vi "SFCS_ChkRoute_ComCode.vi"(5 "URL":string) -> (1 "Status":string)   [LabVIEW 2011]
uses:
  Instance           4 29Saved   SFCS_ChkRoute_ComCode .vi
  Instance           1 29Saved   SFCS_ChkRoute_ComCode .vi
  Instance           2 29Saved   SFCS_ChkRoute_ComCode .vi
  Instance           3 29Saved   SFCS_ChkRoute_ComCode .vi
  Instance           5 29Saved   SFCS_ChkRoute_ComCode .vi
  data/MCSDLL.dll
panel:
  out "軟體版本Software Version":string
  out "Begin time":u32
  out "SFCS System Enable":string
  out "ComCode":string
  out "Category":string
  out "COMCODE":string
  out "STAGE":string
  out "Unit SN":string
  out "USN_Length":i32
  out "SFCS_IP":string
  # "SFCS Check Route"
  # "2014-12-15"
  # "SFCS的網址"
  # "站名"
  # "序號"
  # "訊息"
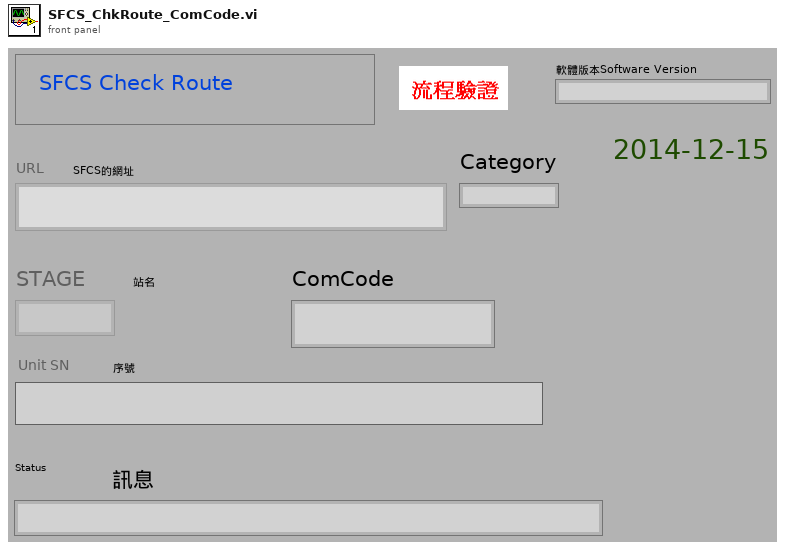
[diagram p1: front panel]
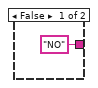
[diagram p5: hidden frame]
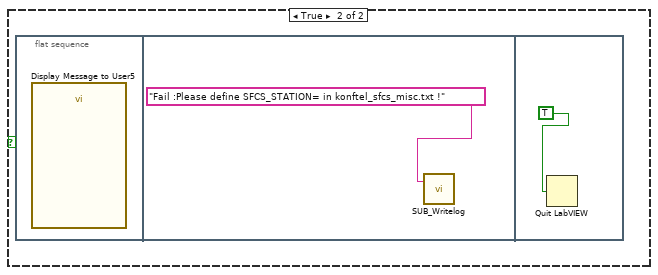
[diagram p7: hidden frame]
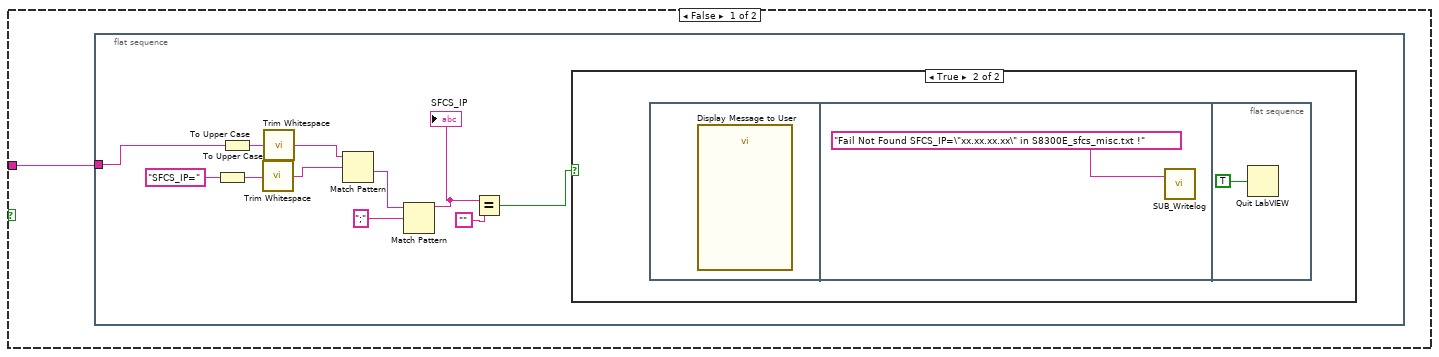
[diagram p9: hidden frame]
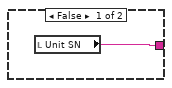
[diagram p11: hidden frame]
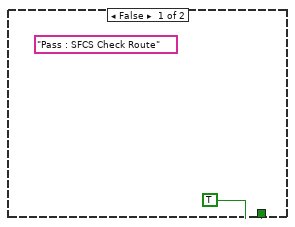
[diagram p12: hidden frame]
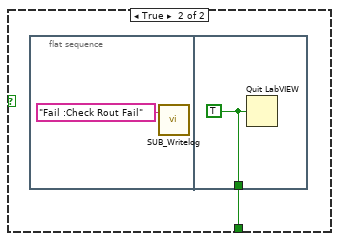
[diagram p13: hidden frame]
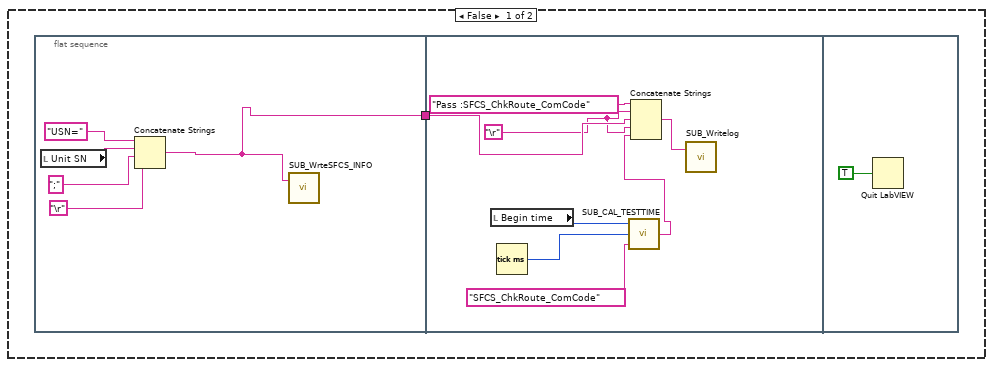
[diagram p14: hidden frame]
diagram:
  n1 = flat-sequence {
    tunnel: [w120] -> w2
    tunnel: [w119] -> w1
    tunnel: w2 -> [w139]
    tunnel: w1 -> [w135]
    frame #0 {
      n2 = Tick Count (ms)() -> (millisecond timer value=→"Begin time":u32)
    }
    frame #1 {
      n3 = call "SUB_SW_Version.vi"() -> ("Current Software Version"=→"軟體版本Software Version":string)  [unwired: 3 in]
      n4 = local write "Unit SN"("") -> ()
    }
    frame #2 {
      n5 = call "SUB_ReadScript_File.vi"("Script FileName"="barcode.log" ("name or relative path")) -> ("text"=w6:string, "error out"=w9:errorcluster)  [unwired: 1 in, 1 out]
      n6 = Unbundle(w9) -> ("code"=w8:i32)  [unwired: 2 out]
      n7 = Equal To 0?(x=w8) -> (x = 0?=w7:bool)
      n8 = case shown="True" w7 {
        tunnel: w6 -> [_ w13]
        frame False {
        }
        frame True {
          n9 = call "SUB_FindSpecificString.vi"("Find this String"="PRODUCT_SN=", "String data"=w13) -> ("before \"; \" string"=w11:string, "Found"=w12:bool)  [unwired: 2 in]
          n10 = case shown="True" w12 {
            tunnel: w11 -> [_ w15]
            frame False {
            }
            frame True {
              n11 = local write "Unit SN"(w15) -> ()
            }
          }
        }
      }
    }
    frame #3 {
      # "Check SFCS Enable in Mojo_script.txt"
      n12 = call "SUB_ReadScript_File.vi"("Script FileName"="S8300E_sfcs_misc.txt") -> ("text"=w21:string, "error out"=w18:errorcluster)  [unwired: 1 in, 1 out]
      n13 = Unbundle By Name(w18) -> ("code"=w19:i32)
      n14 = Equal To 0?(x=w19) -> (x = 0?=w20:bool)
      n15 = case shown="True" w20 {
        tunnel: w21 -> [_ w29]
        tunnel: ["NO" ("before \"; \" string") w27] -> w22
        frame False {
        }
        frame True {
          n16 = call "SUB_FindSpecificString.vi"("Find this String"="SFCS_SYSTEM_ENABLE=", "String data"=w29) -> ("before \"; \" string"=w27:string)  [unwired: 2 in, 1 out]
          "SFCS System Enable" <- w27
        }
      }
      n17 = Equal?(x=w22, y="YES") -> (x = y?=w17:bool)
      n18 = case shown="False" w17 {
        frame False {
          n19 = flat-sequence {
            frame #0 {
              n20 = call "SUB_Writelog.vi"("Pass/Fail"="Done :SFCS_ChkRoute_ComCode by PASS!") -> ()  [unwired: 2 in]
            }
            frame #1 {
              n21 = Quit LabVIEW(quit? (T)=TRUE) -> ()
            }
          }
        }
        frame True {
        }
      }
    }
    frame #4 {
      n22 = call "SUB_DELETE_SpecificFile.vi"("Filename to be  Deleted"="SFCS_INFO.LOG") -> ()  [unwired: 2 in, 1 out]
    }
    frame #5 {
      n23 = call "SUB_ReadScript_File.vi"("Script FileName"="S8300E_sfcs_misc.txt") -> ("text"=w32:string, "error out"=w35:errorcluster)  [unwired: 1 in, 1 out]
      n24 = Unbundle By Name(w35) -> ("code"=w34:i32)
      n25 = Equal To 0?(x=w34) -> (x = 0?=w33:bool)
      n26 = case shown="True" w33 {
        tunnel: w32 -> [_ w36]
        frame False {
        }
        frame True {
          n27 = To Upper Case(1:"SFCS_USNLength=" ("string")) -> (0:w45:string)
          n28 = To Upper Case(1:w36) -> (0:w47:string)
          n29 = call <vilib>:"Trim Whitespace.vi"("string"=w45) -> ("trimmed string"=w43:string)  [unwired: 1 in]
          n30 = call <vilib>:"Trim Whitespace.vi"("string"=w47) -> ("trimmed string"=w46:string)  [unwired: 1 in]
          n31 = Match Pattern(string=w46, regular expression=w43) -> (after substring=w41:string)  [unwired: 1 in, 3 out]
          n32 = Match Pattern(string=w41, regular expression=";") -> (before substring=w38:string)  [unwired: 1 in, 3 out]
          n33 = Equal?(x=w38, y="") -> (x = y?=w39:bool)
          n34 = Decimal String To Number(string=w38) -> (number=→"USN_Length":i32)  [unwired: 2 in, 1 out]
          n35 = case shown="False" w39 {
            tunnel: w36 -> [w51 _]
            frame False {
              n36 = To Upper Case(1:"SFCS_STATION=" ("string")) -> (0:w56:string)
              n37 = To Upper Case(1:w51) -> (0:w58:string)
              n38 = call <vilib>:"Trim Whitespace.vi"("string"=w56) -> ("trimmed string"=w54:string)  [unwired: 1 in]
              n39 = call <vilib>:"Trim Whitespace.vi"("string"=w58) -> ("trimmed string"=w57:string)  [unwired: 1 in]
              n40 = Match Pattern(string=w57, regular expression=w54) -> (after substring=w52:string)  [unwired: 1 in, 3 out]
              n41 = Match Pattern(string=w52, regular expression=";") -> (before substring=w50:string)  [unwired: 1 in, 3 out]
              "STAGE" <- w50
              n42 = Equal?(x=w50, y="") -> (x = y?=w48:bool)
              n43 = case shown="False" w48 {
                frame False {
                }
                frame True {
                  n44 = flat-sequence {
                    frame #0 {
                      n45 = call "Display Message to User5"() -> ()  [unwired: 10 in, 2 out]
                    }
                    frame #1 {
                      n46 = call "SUB_Writelog.vi"("Pass/Fail"="Fail :Please define SFCS_STATION= in konftel_sfcs_misc.txt !") -> ()  [unwired: 2 in]
                    }
                    frame #2 {
                      n47 = Quit LabVIEW(quit? (T)=TRUE) -> ()
                    }
                  }
                }
              }
            }
            frame True {
            }
          }
        }
      }
    }
    frame #6 {
      n48 = call "SUB_ReadScript_File.vi"("Script FileName"="S8300E_sfcs_misc.txt") -> ("text"=w62:string, "error out"=w65:errorcluster)  [unwired: 1 in, 1 out]
      n49 = Unbundle By Name(w65) -> ("code"=w64:i32)
      n50 = Not Equal To 0?(x=w64) -> (x != 0?=w63:bool)
      n51 = case shown="True" w63 {
        tunnel: w62 -> [w66 _]
        frame False {
          n52 = flat-sequence {
            tunnel: w66 -> [w72]
            frame #0 {
              n53 = To Upper Case(1:"SFCS_IP=" ("string")) -> (0:w76:string)
              n54 = To Upper Case(1:w72) -> (0:w77:string)
              n55 = call <vilib>:"Trim Whitespace.vi"("string"=w76) -> ("trimmed string"=w74:string)  [unwired: 1 in]
              n56 = call <vilib>:"Trim Whitespace.vi"("string"=w77) -> ("trimmed string"=w73:string)  [unwired: 1 in]
              n57 = Match Pattern(string=w73, regular expression=w74) -> (after substring=w71:string)  [unwired: 1 in, 3 out]
              n58 = Match Pattern(string=w71, regular expression=";") -> (before substring=w69:string)  [unwired: 1 in, 3 out]
              "SFCS_IP" <- w69
              n59 = Equal?(x=w69, y="") -> (x = y?=w67:bool)
              n60 = case shown="True" w67 {
                frame False {
                }
                frame True {
                  n61 = flat-sequence {
                    frame #0 {
                      n62 = call "Display Message to User"() -> ()  [unwired: 10 in, 2 out]
                    }
                    frame #1 {
                      n63 = call "SUB_Writelog.vi"("Pass/Fail"="Fail Not Found SFCS_IP=\"xx.xx.xx.xx\" in S8300E_sfcs_misc.txt !") -> ()  [unwired: 2 in]
                    }
                    frame #2 {
                      n64 = Quit LabVIEW(quit? (T)=TRUE) -> ()
                    }
                  }
                }
              }
            }
          }
        }
        frame True {
          n65 = flat-sequence {
            frame #0 {
              n66 = call "Display Message to User2"() -> ()  [unwired: 10 in, 2 out]
            }
            frame #1 {
              n67 = call "SUB_Writelog.vi"("Pass/Fail"="Fail S8300E_sfcs_misc.txt  Missing!") -> ()  [unwired: 2 in]
            }
            frame #2 {
              n68 = Quit LabVIEW(quit? (T)=TRUE) -> ()
            }
          }
        }
      }
    }
    frame #7 {
      n69 = local read "SFCS_IP"() -> (w82:string)
      n70 = local write "URL"(w82) -> ()
    }
    frame #8 {
      n71 = while {
        stop <- w84 stop-if-true
        n72 = flat-sequence {
          tunnel: [w88] -> w83
          tunnel: [w92] -> w84
          tunnel: w83 -> [w91]
          frame #0 {
            n73 = local read "Unit SN"() -> (w87:string)
            n74 = String Length(string=w87) -> (length=w86:i32)
            n75 = Equal To 0?(x=w86) -> (x = 0?=w85:bool)
            n76 = case shown="True" w85 {
              tunnel: [w89 w90] -> w88
              frame False {
                n77 = local read "Unit SN"() -> (w89:string)
              }
              frame True {
                n78 = call "Prompt User for Input"() -> ("Unit SN"=w90:string)  [unwired: 17 in, 2 out]
                "Unit SN" <- w90
              }
            }
          }
          frame #1 {
            n79 = local read "STAGE"() -> (w103:string)
            n80 = dll-call lib="D:/S8300E_Project/data/MCSDLL.dll" fn="SFCS_CheckRoute"("URL"="URL", "SN"=w91, "Stage"=w103) -> (w94:string)  [unwired: 6 in, 2 out]
            "Status" <- w94
            n81 = To Upper Case(1:"OK" ("string")) -> (0:w100:string)
            n82 = To Upper Case(1:w94) -> (0:w102:string)
            n83 = call <vilib>:"Trim Whitespace.vi"("string"=w100) -> ("trimmed string"=w97:string)  [unwired: 1 in]
            n84 = call <vilib>:"Trim Whitespace.vi"("string"=w102) -> ("trimmed string"=w101:string)  [unwired: 1 in]
            n85 = Match Pattern(string=w101, regular expression=w97) -> (match substring=w98:string)  [unwired: 1 in, 3 out]
            n86 = Not Equal?(x=w98, y=w97) -> (x != y?=w96:bool)
            n87 = Concatenate Strings("系統訊息" ("string"), w94) -> (w93:string)
            n88 = case shown="True" w96 {
              tunnel: w93 -> [_ w111]
              tunnel: [TRUE w110] -> w92
              frame False {
                (unwired) "Pass : SFCS Check Route" ("Pass/Fail")
              }
              frame True {
                n89 = call "SUB_YESNO.vi"("Debug View"=w111, "Status"="網路線有插好 ?") -> ("yes/no"=w108:enum32{"No Selection", "Yes", "No", "None"})  [unwired: 1 in]
                n90 = Equal?(x=w108, y=enum32{"No Selection", "Yes", "No", "None"}."No") -> (x = y?=w106:bool)
                n91 = case shown="False" w106 {
                  tunnel: [w112 w115] -> w110
                  frame False {
                    n92 = flat-sequence {
                      tunnel: [FALSE] -> w112
                      frame #0 {
                        n93 = local write "Unit SN"("") -> ()
                      }
                      frame #1 {
                      }
                    }
                  }
                  frame True {
                    n94 = flat-sequence {
                      tunnel: [w117] -> w115
                      frame #0 {
                        n95 = call "SUB_Writelog.vi"("Pass/Fail"="Fail :Check Rout Fail") -> ()  [unwired: 2 in]
                      }
                      frame #1 {
                        w117 = TRUE ("quit? (T)")
                        n96 = Quit LabVIEW(quit? (T)=w117) -> ()
                      }
                    }
                  }
                }
              }
            }
          }
        }
      }
    }
    frame #9 {
      # "c"
      n97 = call "SUB_ReadScript_File.vi"("Script FileName"="S8300E_sfcs_misc.txt") -> ("text"=w128:string)  [unwired: 1 in, 2 out]
      n98 = To Upper Case(1:"SFCS_Category=" ("string")) -> (0:w123:string)
      n99 = To Upper Case(1:"SFCS_COMCODE=" ("string")) -> (0:w132:string)
      n100 = To Upper Case(1:w128) -> (0:w133:string)
      n101 = call <vilib>:"Trim Whitespace.vi"("string"=w123) -> ("trimmed string"=w122:string)  [unwired: 1 in]
      n102 = call <vilib>:"Trim Whitespace.vi"("string"=w132) -> ("trimmed string"=w131:string)  [unwired: 1 in]
      n103 = call <vilib>:"Trim Whitespace.vi"("string"=w133) -> ("trimmed string"=w124:string)  [unwired: 1 in]
      n104 = Match Pattern(string=w124, regular expression=w131) -> (after substring=w129:string)  [unwired: 1 in, 3 out]
      n105 = Match Pattern(string=w124, regular expression=w122) -> (after substring=w125:string)  [unwired: 1 in, 3 out]
      n106 = Match Pattern(string=w129, regular expression=";") -> (before substring=w119:string)  [unwired: 1 in, 3 out]
      "COMCODE" <- w119
      n107 = Match Pattern(string=w125, regular expression=";") -> (before substring=w120:string)  [unwired: 1 in, 3 out]
      "Category" <- w120
    }
    frame #10 {
      n108 = local read "Unit SN"() -> (w141:string)
      n109 = local read "URL"() -> (w142:string)
      n110 = local read "STAGE"() -> (w140:string)
      n111 = dll-call lib="D:/S8300E_Project/data/MCSDLL.dll" fn="SFCS_GetMOInfo"("URL"=w142, "SN"=w141, "Stage"=w140, "Category"=w139) -> (w137:string)  [unwired: 7 in, 2 out]
      n112 = To Upper Case(1:w137) -> (0:w138:string)
      n113 = call <vilib>:"Trim Whitespace.vi"("string"=w138) -> ("trimmed string"=w136:string)  [unwired: 1 in]
      "ComCode" <- w136
      n114 = Not Equal?(x=w136, y=w135) -> (x != y?=w134:bool)
      n115 = case shown="True" w134 {
        frame False {
          n116 = flat-sequence {
            tunnel: [w144] -> w143
            tunnel: w143 -> [w152]
            frame #0 {
              n117 = local read "Unit SN"() -> (w146:string)
              n118 = Concatenate Strings("USN=" ("string"), w146, ";", "\r") -> (w144:string)
              n119 = call "SUB_WrteSFCS_INFO.vi"("Pass/Fail"=w144) -> ()  [unwired: 2 in]
            }
            frame #1 {
              w151 = "\r"
              n120 = local read "Begin time"() -> (w156:u32)
              n121 = Tick Count (ms)() -> (millisecond timer value=w155:u32)
              n122 = call "SUB_CAL_TESTTIME.vi"("Test Item name"="SFCS_ChkRoute_ComCode", "Stop tick time"=w155, "Start tick time"=w156) -> ("Test Time output"=w150:string)  [unwired: 2 in]
              n123 = Concatenate Strings("Pass :SFCS_ChkRoute_ComCode" ("Pass/Fail"), w151, w152, w151, w150) -> (w149:string)
              n124 = call "SUB_Writelog.vi"("Pass/Fail"=w149) -> ()  [unwired: 2 in]
            }
            frame #2 {
              n125 = Quit LabVIEW(quit? (T)=TRUE) -> ()
            }
          }
        }
        frame True {
          n126 = flat-sequence {
            frame #0 {
              n127 = call "Display Message to User7"() -> ()  [unwired: 10 in, 2 out]
            }
            frame #1 {
              n128 = call "SUB_Writelog.vi"("Pass/Fail"="Fail  :ComCode not Match or SFCS Problem !") -> ()  [unwired: 2 in]
            }
            frame #2 {
              n129 = Quit LabVIEW(quit? (T)=TRUE) -> ()
            }
          }
        }
      }
    }
  }
